vi "Dummy run form.vi"(0 "Stack in":refnum<class "Stack.lvclass">, 1 "Adhesive type":string, 2 "Baselayer thickness for glue dispense":dbl, 5 "Position":dbl, 7 "Module Type":string, 9 "Module?":bool, 11 "error in (no error)":errorcluster, 13 "ROC version":string) -> (4 "Stack out":refnum<class "Stack.lvclass">, 15 "error out":errorcluster)   [LabVIEW 2021, in "Stack.lvclass"]
uses:
  Stack.lvclass
  Stack.lvclass/Stack.ctl
panel:
  out "Resolution":string
  out "Geometry":string
  out "BP Type":string
  out "Sensor thickness":string
  out "Date":string
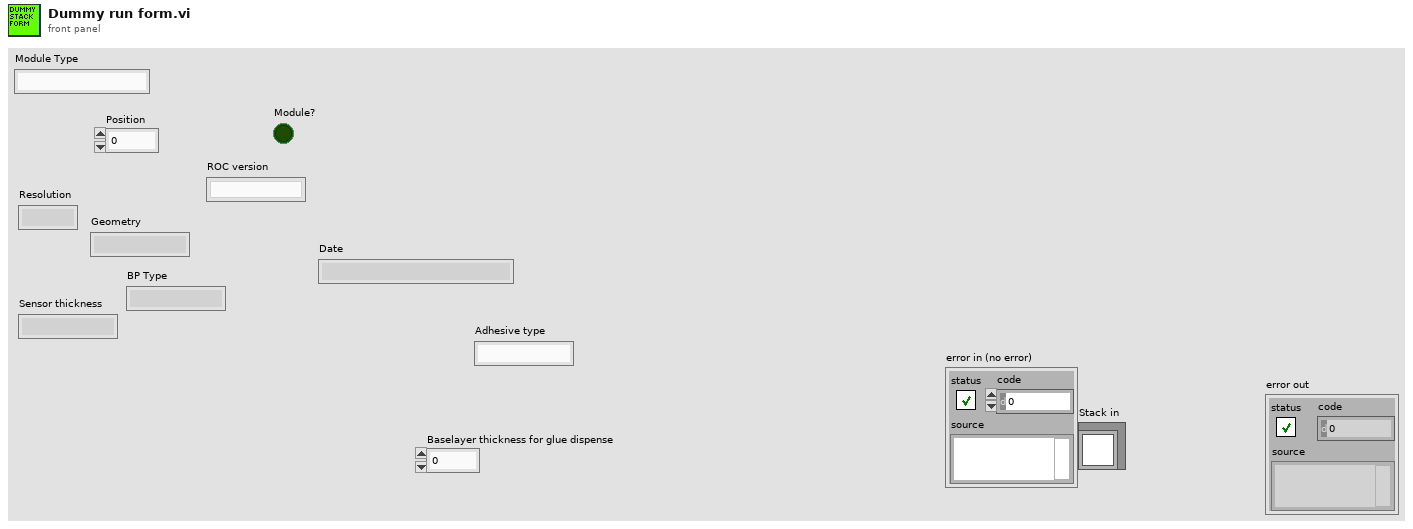
[diagram p1: front panel]
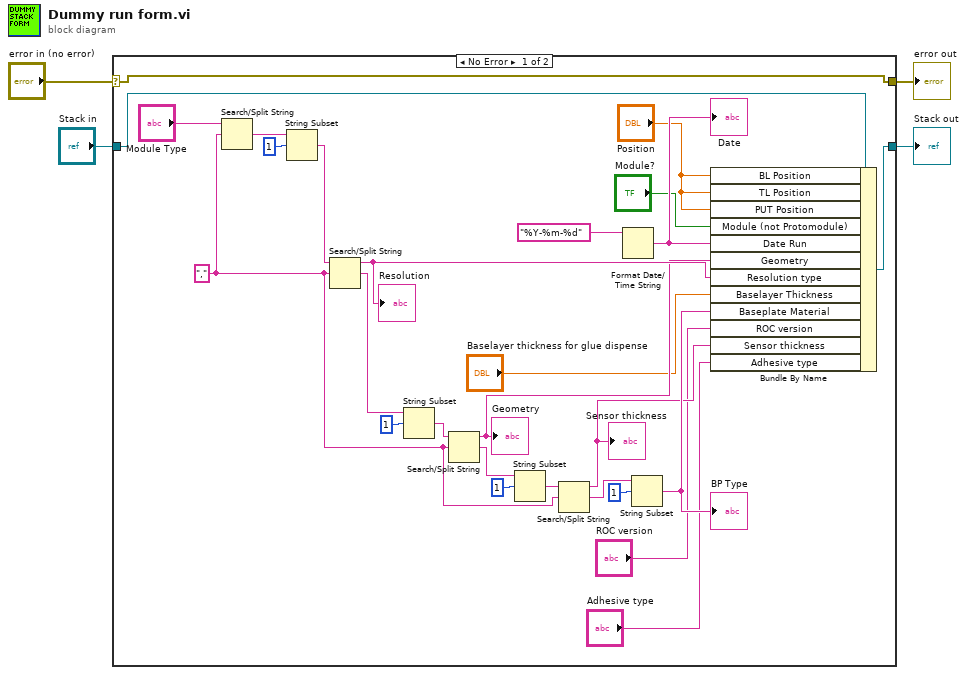
[diagram p0: block diagram]
diagram:
  n1 = case shown="No Error" "error in (no error)" {
    selector: "error in (no error)" -> [w31 w33]
    tunnel: [w31 w33] -> w3
    tunnel: [w29 w32] -> w1
    tunnel: "Stack in" -> [w30 w32]
    frame No Error {
      w21 = "," ("search string/char (-)")
      n2 = Search/Split String(string="Module Type", search string/char (-)=w21) -> (match + rest of string=w27:string)  [unwired: 1 in, 2 out]
      n3 = String Subset(string=w27, offset (0)=1) -> (substring=w26:string)  [unwired: 1 in]
      n4 = Search/Split String(string=w26, search string/char (-)=w21) -> (substring before match=w22:string, match + rest of string=w25:string)  [unwired: 1 in, 1 out]
      "Resolution" <- w22
      n5 = String Subset(string=w25, offset (0)=1) -> (substring=w15:string)  [unwired: 1 in]
      n6 = Search/Split String(string=w15, search string/char (-)=w21) -> (substring before match=w12:string, match + rest of string=w19:string)  [unwired: 1 in, 1 out]
      "Geometry" <- w12
      n7 = String Subset(string=w19, offset (0)=1) -> (substring=w20:string)  [unwired: 1 in]
      n8 = Search/Split String(string=w20, search string/char (-)=w21) -> (substring before match=w13:string, match + rest of string=w18:string)  [unwired: 1 in, 1 out]
      "Sensor thickness" <- w13
      n9 = Format Date/Time String(time format string (%c)="%Y-%m-%d") -> (date/time string=w10:string)  [unwired: 2 in]
      "Date" <- w10
      n10 = String Subset(string=w18, offset (0)=1) -> (substring=w14:string)  [unwired: 1 in]
      "BP Type" <- w14
      n11 = Bundle By Name(cluster=w30, "BL Position"="Position", "TL Position"="Position", "PUT Position"="Position", "Module (not Protomodule)"="Module?", "Date Run"=w10, "Geometry"=w12, "Resolution type"=w22, "Baselayer Thickness"="Baselayer thickness for glue dispense", "Baseplate Material"=w14, "ROC version"="ROC version", "Sensor thickness"=w13, "Adhesive type"="Adhesive type") -> (w29:refnum<class "Stack.lvclass">)
    }
    frame Error {
    }
  }
  "error out" <- w3
  "Stack out" <- w1
